vi "Refresh Waveform.vi"(8 "error in":errorcluster, 10 "Waveform":waveform(dbl)[](array[waveform]), 11 "Report Viewer in":refnum<class "Report Viewer.lvclass">) -> (0 "error out":errorcluster, 3 "Report Viewer out":refnum<class "Report Viewer.lvclass">)   [LabVIEW 2019, in "Report Viewer.lvlib" / "Report Viewer.lvclass"]
uses:
  Library/Report Viewer.lvclass
  Library/Report Viewer.lvclass/Report Viewer.ctl
  <vilib>/Waveform/WDTOps.llb/WDT Get Waveform Time Array DBL.vi
panel:
  out "XY Graph":cluster{"X array":timestamp[], "Y":dbl[]}[](graph)
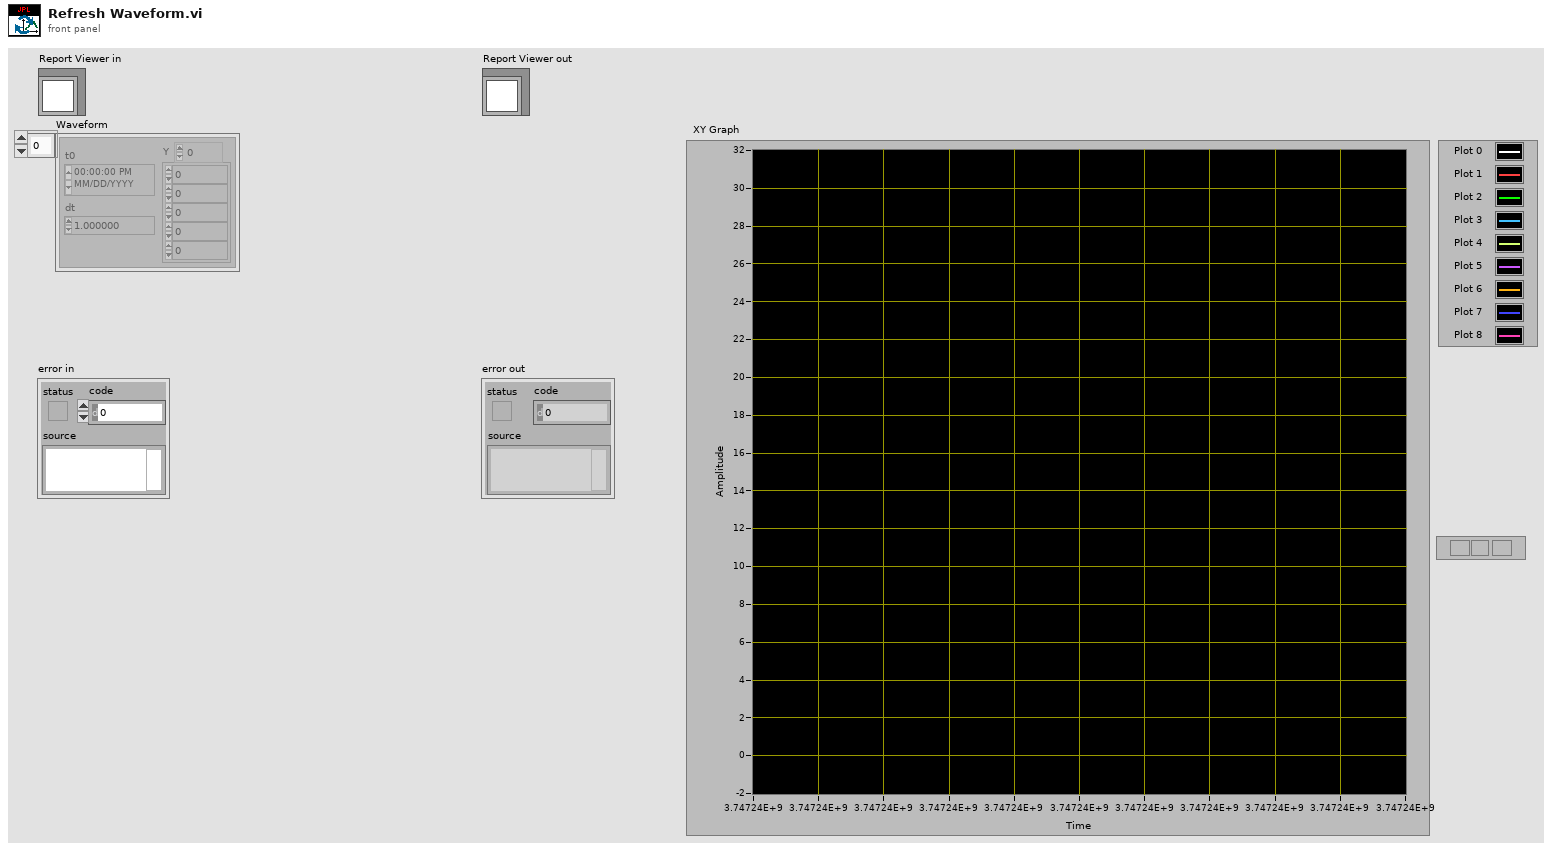
[diagram p1: front panel]
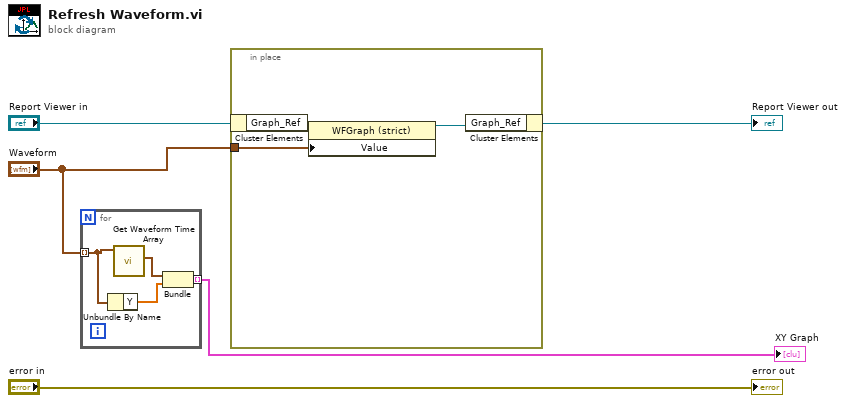
[diagram p0: block diagram]
diagram:
  n1 = for {
    tunnel: "Waveform" -> [w9] mode=indexing
    tunnel: [w6] -> w1 mode=indexing
    n2 = Unbundle By Name(w9) -> ("Y"=w7:dbl[])
    n3 = call-poly <vilib>:"Get Waveform Time Array.vi"("waveform in"=w9) -> ("X array"=w8:timestamp[])  [unwired: 9 in, 1 out]
    n4 = Bundle("X array"=w8, "Y"=w7) -> (w6:cluster{"X array":timestamp[], "Y":dbl[]})  [unwired: 1 in]
  }
  "XY Graph" <- w1
  n5 = in-place {
    in-place-border: "Waveform" -> [w10]
    n6 = in-place-cluster #1("Report Viewer in") -> ("Graph_Ref"=w12:refnum<vi>)
    n7 = property class="WFGraph (strict)"(reference=w12, "Value"=w10) -> (reference out=w11:refnum<vi>)  [unwired: 1 in, 1 out]
    n8 = in-place-cluster #1("Graph_Ref"=w11) -> (→"Report Viewer out":refnum<class "Report Viewer.lvclass">)
  }
  "error out" <- "error in"
